vi "Load data.vi"(0 "reference in":refnum<class "TDMS_DataHandler.lvclass">, 2 "TDMS Filepath":path, 5 "error in (no error)":errorcluster) -> (13 "size (in bytes)":i64=37399506 format="%.0p", 14 "reference out":refnum<class "TDMS_DataHandler.lvclass">, 15 "Channel name(s)":string[](array[string]), 16 "Channels out":waveform(dbl)[](array[waveform]), 17 "Group metadata":T1, 19 "error out":errorcluster)   [LabVIEW 2019, in "TDMS_DataHandler.lvclass"]
uses:
  TDMS_DataHandler.lvclass
  Fcurve Meta data.ctl
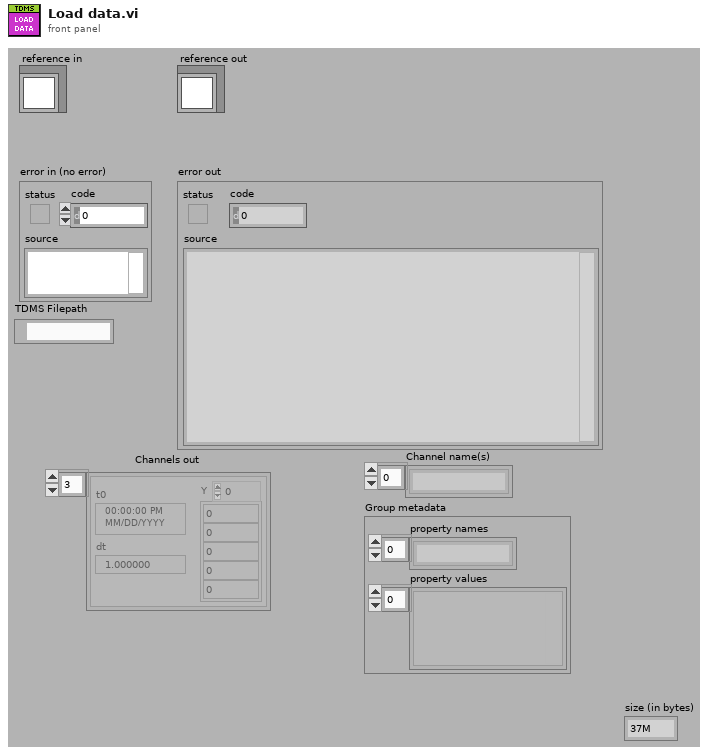
[diagram p1: front panel]
types:
  T1 = typedef "TDMS_DataHandler.lvclass/Fcurve Meta data.ctl" = cluster{"property names":string[], "property values":variant[]}
  T2 = cluster{"property names":string[], "property values":variant[]}
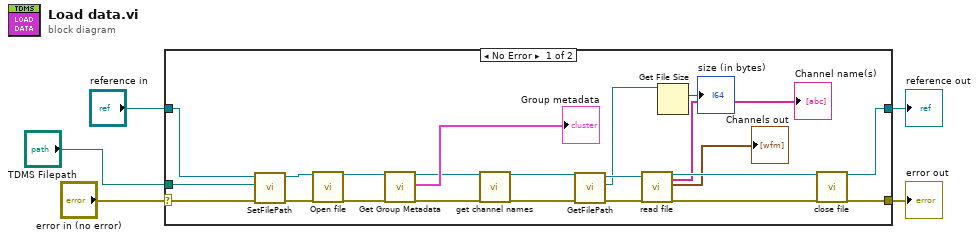
[diagram p0: block diagram]
diagram:
  n1 = case shown="No Error" "error in (no error)" {
    selector: "error in (no error)" -> [w8 w29]
    tunnel: [w25 w29] -> w4
    tunnel: [w23 w28] -> w2
    tunnel: "reference in" -> [w10 w28]
    tunnel: "TDMS Filepath" -> [w6 _]
    frame No Error {
      n2 = call-dynamic "SetFilePath.vi"("error in (no error)"=w8, "Filepath"=w6, "reference in"=w10) -> ("error out"=w7:errorcluster, "reference out"=w9:refnum<class "TDMS_DataHandler.lvclass">)  [unwired: 7 in]
      n3 = call-dynamic "Open file.vi"("reference in"=w9, "error in (no error)"=w7) -> ("reference out"=w22:refnum<class "TDMS_DataHandler.lvclass">, "error out"=w21:errorcluster)  [unwired: 15 in, 1 out]
      n4 = call-dynamic "Get Group Metadata.vi"("reference in"=w22, "error in (no error)"=w21) -> ("reference out"=w14:refnum<class "TDMS_DataHandler.lvclass">, "Tdms metadata out"=→"Group metadata":T2, "error out"=w12:errorcluster)  [unwired: 15 in]
      n5 = call-dynamic "get channel names.vi"("reference in"=w14, "error in (no error)"=w12) -> ("reference out"=w13:refnum<class "TDMS_DataHandler.lvclass">, "error out"=w11:errorcluster)  [unwired: 14 in, 2 out]
      n6 = call-dynamic "GetFilePath.vi"("error in (no error)"=w11, "reference in"=w13) -> ("error out"=w17:errorcluster, "Filepath"=w15:path, "reference out"=w18:refnum<class "TDMS_DataHandler.lvclass">)  [unwired: 7 in]
      n7 = call-dynamic "read file.vi"("reference in"=w18, "error in (no error)"=w17) -> ("reference out"=w26:refnum<class "TDMS_DataHandler.lvclass">, "Channel name(s)"=→"Channel name(s)":string[], "Data out"=→"Channels out":waveform(dbl)[], "error out"=w27:errorcluster)  [unwired: 13 in, 1 out]
      n8 = Get File Size(file=w15) -> (size (in bytes)=→"size (in bytes)":i64)  [unwired: 1 in, 2 out]
      n9 = call-dynamic "close file.vi"("reference in"=w26, "error in (no error)"=w27) -> ("reference out"=w23:refnum<class "TDMS_DataHandler.lvclass">, "error out"=w25:errorcluster)  [unwired: 16 in]
    }
    frame Error {
    }
  }
  "error out" <- w4
  "reference out" <- w2
